vi "Vision Research Phantom Series PhLV Progress2.vi"(0 "Continue":refnum<vi>, 1 "Progress":refnum<vi>, 5 "error in (no error)":errorcluster, 7 "CallID":u32) -> (19 "error out":errorcluster)   [LabVIEW 2013, in "VRI.lvlib"]
uses:
  VRI.lvlib
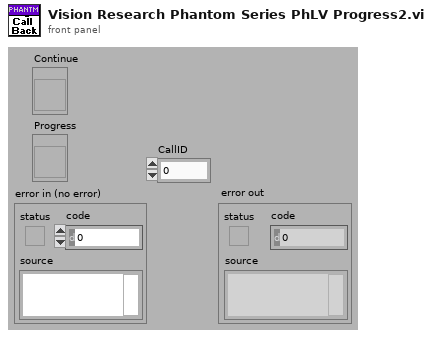
[diagram p1: front panel]
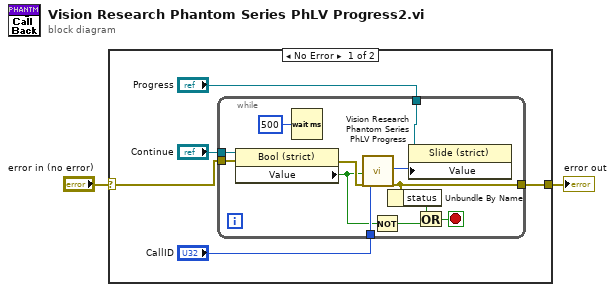
[diagram p0: block diagram]
diagram:
  n1 = case shown="No Error" "error in (no error)" {
    selector: "error in (no error)" -> [w3 w20]
    tunnel: [w5 w20] -> w2
    frame No Error {
      n2 = while {
        tunnel: "CallID" -> [w19]
        tunnel: [w13] -> w5
        tunnel: "Continue" -> [w17]
        tunnel: "Progress" -> [w11]
        tunnel: w3 -> [w9]
        stop <- w14 stop-if-true
        n3 = property class="Bool (strict)"(reference=w17, error in=w9) -> (error out=w16:errorcluster, "Value"=w15:bool)  [unwired: 1 out]
        n4 = Wait (ms)(milliseconds to wait=u32 500) -> ()  [unwired: 1 out]
        n5 = call "Vision Research Phantom Series PhLV Progress.vi"("Continue"=w15, "Error In (no error)"=w16, "CallID"=w19) -> ("pPercent"=w10:u32, "Error Out"=w13:errorcluster)  [unwired: 15 out]
        n6 = Not(x=w15) -> (.not. x?=w8:bool)
        n7 = Unbundle By Name(w13) -> ("status"=w12:bool)
        n8 = property class="Slide (strict)"(reference=w11, "Value"=w10) -> ()  [unwired: 1 in, 2 out]
        n9 = Or(x=w12, y=w8) -> (x .or. y?=w14:bool)
      }
    }
    frame Error {
    }
  }
  "error out" <- w2
